vi "Update.vi"(8 "error in (no error)":errorcluster, 11 "Cat in":refnum<class "Cat.lvclass">) -> (0 "error out":errorcluster, 2 "Variant":variant, 3 "Cat out":refnum<class "Cat.lvclass">)   [LabVIEW 2013, in "Cat.lvclass"]
uses:
  Cat.lvclass
  Observer.lvclass/Observer.lvclass
  Cat.lvclass/Cat.ctl
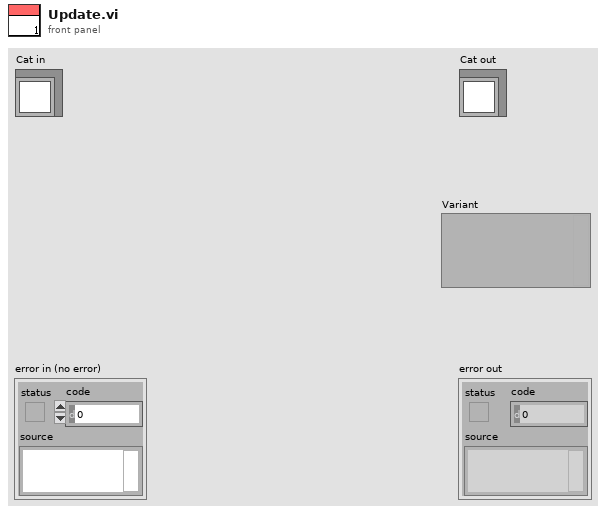
[diagram p1: front panel]
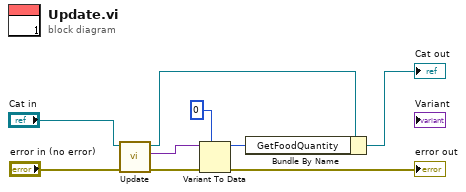
[diagram p0: block diagram]
diagram:
  n1 = call-parent "Update.vi"("error in (no error)"="error in (no error)", "Observer in"="Cat in") -> ("error out"=w4:errorcluster, "Variant"=w6:variant, "Observer out"=w7:refnum<class "Cat.lvclass">)  [unwired: 7 in]
  n2 = Variant To Data(error in=w4, type=0, Variant=w6) -> (data=w2:i32, error out=→"error out":errorcluster)
  n3 = Bundle By Name(cluster=w7, "GetFoodQuantity"=w2) -> (→"Cat out":refnum<class "Cat.lvclass">)
